vi "CCP_tcp_server.vi"(5 "timeout":i32=1000, 6 "value":refnum<vi>[](array[refnum]), 7 "port":u16=10000, 8 "error_in":errorcluster, 11 "conn_id_in":refnum<k5>) -> (0 "error_out":errorcluster, 3 "conn_id_out":refnum<k5>, 4 "status":string)   [LabVIEW 2019]
panel:
  in  "clear_error":bool=TRUE
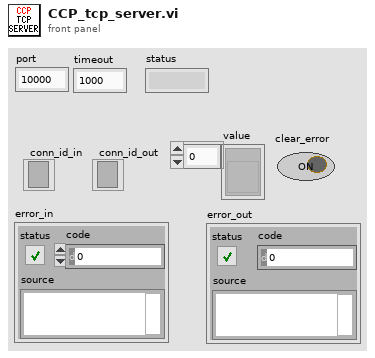
[diagram p1: front panel]
types:
  T1 = enum16{"Standard", "Buffered", "CRLF", "Immediate"}
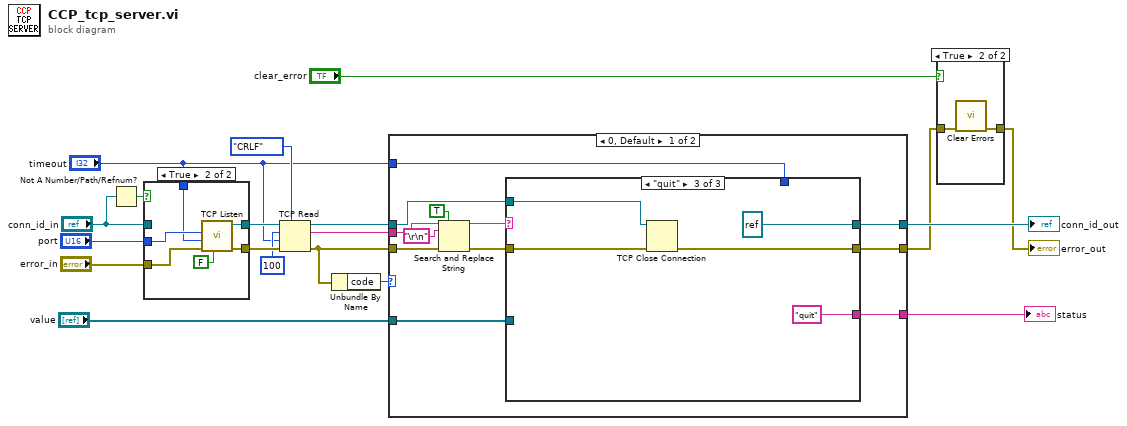
[diagram p0: block diagram]
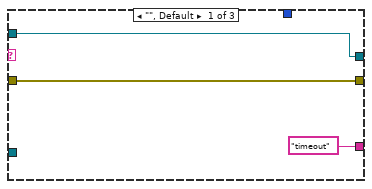
[diagram p3: hidden frame]
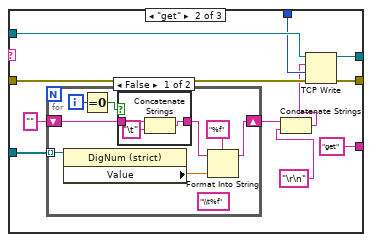
[diagram p4: hidden frame]
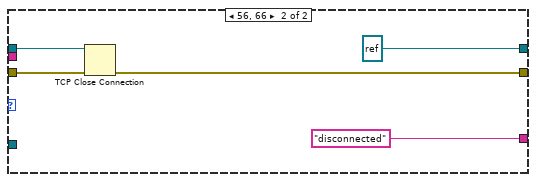
[diagram p6: hidden frame]
diagram:
  n1 = Not A Number/Path/Refnum?(number/path/refnum="conn_id_in") -> (NaN/Path/Refnum?=w19:bool)
  n2 = case shown="True" w19 {
    tunnel: [w21 w27] -> w16
    tunnel: "conn_id_in" -> [w21 _]
    tunnel: "port" -> [_ w26]
    tunnel: "timeout" -> [_ w25]
    tunnel: [w20 w23] -> w14
    tunnel: "error_in" -> [w20 w22]
    frame False {
    }
    frame True {
      n3 = call <vilib>:"TCP Listen.vi"("resolve remote address (T)"=FALSE, "error in (no error)"=w22, "timeout ms (wait forever: -1)"=w25, "port"=w26) -> ("error out"=w23:errorcluster, "connection ID"=w27:refnum<k5>)  [unwired: 3 in, 3 out]
    }
  }
  n4 = TCP Read(connection ID=w16, bytes to read=100, error in (no error)=w14, 7:T1."CRLF" ("mode (standard)"), 9:"timeout") -> (connection ID out=w10:refnum<k5>, data out=w11:string, error out=w6:errorcluster)
  n5 = Unbundle By Name(w6) -> ("code"=w5:i32)
  n6 = case shown="0, Default" w5 {
    tunnel: w11 -> [w39 _]
    tunnel: w10 -> [w35 w72]
    tunnel: [w33 w71] -> w3
    tunnel: "timeout" -> [w32 _]
    tunnel: [w31 refnum<k5> refnum ("conn_id 2")] -> w8
    tunnel: [w30 "disconnected"] -> w7
    tunnel: w6 -> [w29 w73]
    tunnel: "value" -> [w28 _]
    frame 0, Default {
      n7 = Search and Replace String(replace all?=TRUE ("replace all? (F)"), input string=w39, search string="\r\n", error in=w29) -> (result string=w36:string, error out=w34:errorcluster)  [unwired: 4 in, 2 out]
      n8 = case shown="\"quit\"" w36 {
        tunnel: w35 -> [w42 w51 w70]
        tunnel: w34 -> [w41 w52 w69]
        tunnel: [w42 w50 refnum<k5> refnum ("conn_id 2")] -> w31
        tunnel: [w41 w53 w67] -> w33
        tunnel: w32 -> [_ w49 _]
        tunnel: ["timeout" "get" "quit"] -> w30
        tunnel: w28 -> [_ w47 _]
        frame "", Default {
        }
        frame "get" {
          n9 = for {
            tunnel: w47 -> [w59] mode=indexing
            shift-right: [w60] -> w45
            shift-left: "" -> [w56]
            i -> [w58]
            (unwired) "\\t%f" ("f")
            n10 = property on="Property Node" class="DigNum (strict)"(reference=w59) -> ("Value"=w61:dbl)  [unwired: 1 in, 2 out]
            n11 = Equal To 0?(x=w58) -> (x = 0?=w57:bool)
            n12 = case shown="False" w57 {
              tunnel: w56 -> [w64 w65]
              tunnel: [w62 w65] -> w55
              frame False {
                n13 = Concatenate Strings(w64, "\t" ("string")) -> (w62:string)
              }
              frame True {
              }
            }
            n14 = Format Into String(format string="%f", initial string=w55, w61) -> (resulting string=w60:string)  [unwired: 1 in, 1 out]
          }
          n15 = Concatenate Strings(w45, "\r\n" ("format string")) -> (w43:string)
          n16 = TCP Write(connection ID=w51, data in=w43, error in (no error)=w52, 9:w49) -> (connection ID out=w50:refnum<k5>, error out=w53:errorcluster)  [unwired: 1 out]
        }
        frame "quit" {
          n17 = TCP Close Connection(connection ID=w70, error in (no error)=w69) -> (error out=w67:errorcluster)  [unwired: 1 in, 1 out]
        }
      }
    }
    frame 56, 66 {
      n18 = TCP Close Connection(connection ID=w72, error in (no error)=w73) -> (error out=w71:errorcluster)  [unwired: 1 in, 1 out]
    }
  }
  "status" <- w7
  "conn_id_out" <- w8
  n19 = case shown="True" "clear_error" {
    tunnel: w3 -> [w76 w78]
    tunnel: [w76 w77] -> w2
    frame False {
    }
    frame True {
      n20 = call <vilib>:"Clear Errors.vi"("error in (no error)"=w78) -> ("error out"=w77:errorcluster)  [unwired: 5 in, 1 out]
    }
  }
  "error_out" <- w2
